vi "Seconds Breakdown.vi"() -> ()   [LabVIEW 2014]
panel:
  out "Seconds":dbl
  out "Minutes":dbl
  out "Hours":dbl
  in  "Total Time in Seconds":dbl
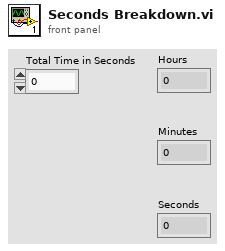
[diagram p1: front panel]
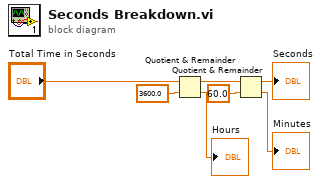
[diagram p0: block diagram]
diagram:
  n1 = Quotient & Remainder(x="Total Time in Seconds", y=3600.0) -> (x-y*floor(x/y)=w5:dbl, floor(x/y)=→"Hours":dbl)
  n2 = Quotient & Remainder(x=w5, y=60.0) -> (x-y*floor(x/y)=→"Seconds":dbl, floor(x/y)=→"Minutes":dbl)
